vi "DIAdem Request Restart.vi"(8 "error in (no error)":errorcluster, 9 "Wait For Completion? (f)":bool, 10 "Override? (f)":bool) -> (0 "error out":errorcluster)   [LabVIEW 2011]
uses:
  DIAdem Daemon Queue.ctl
  DIAdem Daemon Script Type.ctl
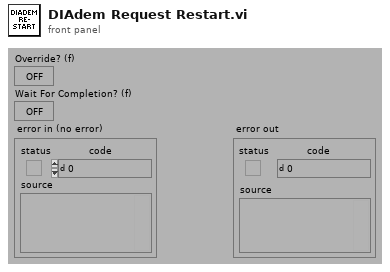
[diagram p1: front panel]
types:
  T1 = typedef "DIAdem Daemon Queue.ctl" = cluster{"Report Template TDM":path, "Report Processor VBS":path, "Report Path PDF":path, "Report Script Params":string, "Username":string, "Script Type":T2, "Report Query Params":string, "Client Machine":string, "Print on Client?":bool, "Response Queue Name":string, "Script Variables":string[], "Start Request Time":timestamp, "Wait?":bool}
  T2 = typedef "DIAdem Daemon Script Type.ctl" = enum16{"Report", "Query", "Script", "Datasheet", "Append", "Restart", "Stop"}
  T3 = typedef "LVDateTimeRec.ctl" = cluster{"fractional second":dbl, "second":i32, "minute":i32, "hour":i32, "day of month":i32, "month":i32, "year":i32, "day of week":i32, "day of year":i32, "DST":i32}
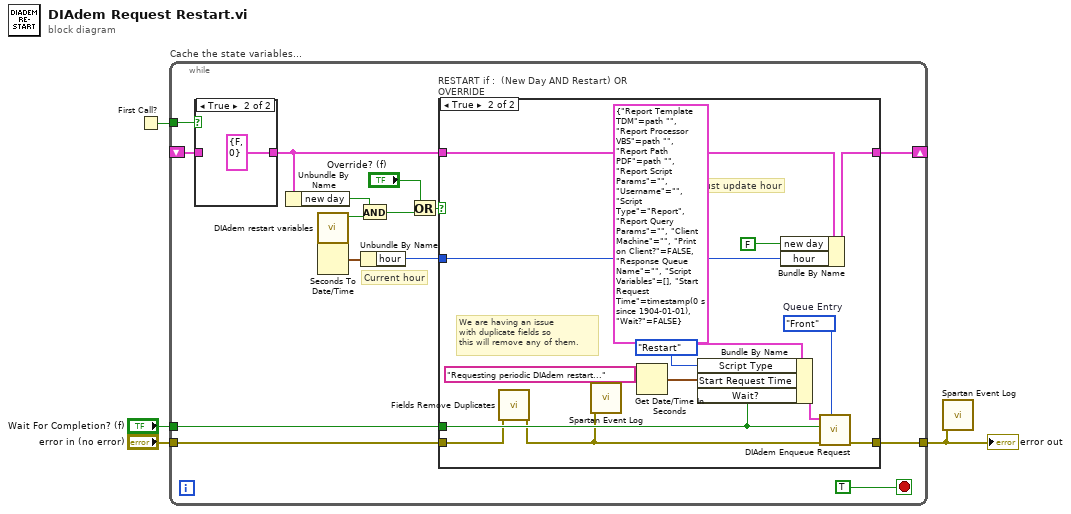
[diagram p0: block diagram]
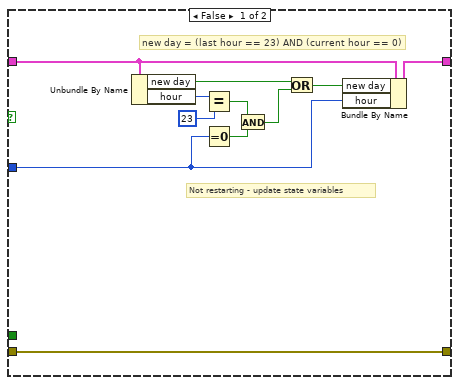
[diagram p3: hidden frame]
diagram:
  n1 = First Call?() -> (First Call?: T/F=w2:bool)
  n2 = while "Cache the state variables..." {
    tunnel: "error in (no error)" -> [w19]
    tunnel: [w16] -> w3
    shift-right: [w9] -> _
    shift-left: _ -> [w6]
    tunnel: w2 -> [w8]
    tunnel: "Wait For Completion? (f)" -> [w5]
    stop <- TRUE stop-if-true
    # "Current hour"
    n3 = case shown="True" w8 {
      tunnel: [w20 cluster{"new day":bool, "hour":i32} {"new day"=FALSE, "hour"=0} ("state")] -> w7
      tunnel: w6 -> [w20 _]
      frame False {
      }
      frame True {
      }
    }
    n4 = Unbundle By Name(w7) -> ("new day"=w12:bool)
    n5 = call "DIAdem restart variables.vi"() -> ("Needs Restart?"=w18:bool)  [unwired: 11 out]
    n6 = Seconds To Date/Time() -> (date time rec=w15:T3)  [unwired: 2 out]
    n7 = And(x=w12, y=w18) -> (x .and. y?=w11:bool)
    n8 = Unbundle By Name(w15) -> ("hour"=w14:i32)
    n9 = Or(x="Override? (f)", y=w11) -> (x .or. y?=w17:bool)
    n10 = case "RESTART if :  (New Day AND Restart) OR OVERRIDE" shown="True" w17 {
      tunnel: [w32 w42] -> w16
      tunnel: w19 -> [w32 w34]
      tunnel: [w31 w38] -> w9
      tunnel: w7 -> [w30 w39]
      tunnel: w14 -> [w29 w36]
      tunnel: w5 -> [_ w35]
      frame False {
        # "Not restarting - update state variables"
        # "new day = (last hour == 23) AND (current hour == 0)"
        n11 = Unbundle By Name(w30) -> ("new day"=w24:bool, "hour"=w25:i32)
        n12 = Equal?(x=w25, y=23) -> (x = y?=w27:bool)
        n13 = Equal To 0?(x=w29) -> (x = 0?=w28:bool)
        n14 = And(x=w27, y=w28) -> (x .and. y?=w23:bool)
        n15 = Or(x=w24, y=w23) -> (x .or. y?=w22:bool)
        n16 = Bundle By Name(cluster=w30, "new day"=w22, "hour"=w29) -> (w31:cluster{"new day":bool, "hour":i32})
      }
      frame True {
        w43 = enum16{"Front", "Back"}."Front"  # Queue Entry
        # "We are having an issue\nwith duplicate fields so\nthis will remove any of them."
        # "Restarting - just update hour"
        n17 = call "Fields Remove Duplicates.vi"("error in (no error)"=w34) -> ("error out"=w33:errorcluster)  [unwired: 9 in, 1 out]
        n18 = call "Spartan Event Log.vi"("error in (no error)"=w33, "message (\"\")"="Requesting periodic DIAdem restart..." ("message (\"\")")) -> ()  [unwired: 3 in, 4 out]
        n19 = Get Date/Time In Seconds() -> (seconds since 1Jan1904=w44:timestamp)
        n20 = Bundle By Name(cluster=T1 {"Report Template TDM"=path "", "Report Processor VBS"=path "", "Report Path PDF"=path "", "Report Script Params"="", "Username"="", "Script Type"=enum."Report", "Report Query Params"="", "Client Machine"="", "Print on Client?"=FALSE, "Response Queue Name"="", "Script Variables"=[], "Start Request Time"=timestamp(0 s since 1904-01-01), "Wait?"=FALSE} ("DD_Report"), "Script Type"=DIAdem_Daemon_Script_Type."Restart", "Start Request Time"=w44, "Wait?"=w35) -> (w45:T1)
        n21 = Bundle By Name(cluster=w39, "new day"=FALSE, "hour"=w36) -> (w38:cluster{"new day":bool, "hour":i32})
        n22 = call "DIAdem Enqueue Request.vi"("Queue Entry"=w43, "error in (no error)"=w33, "Wait for Completion? (f)"=w35, "DD_Report"=w45) -> ("error out"=w42:errorcluster)  [unwired: 1 in, 6 out]
      }
    }
  }
  "error out" <- w3
  n23 = call "Spartan Event Log.vi"("error in (no error)"=w3) -> ()  [unwired: 4 in, 4 out]
